vi "Calculate Analyte Yield.vi"(10 "Max Concentration":dbl, 11 "Peaks":string[][](array[string])) -> (3 "Yield out":dbl)   [LabVIEW 2020, in "Waters Patrol UPLC Report Parser.lvlib"]
uses:
  Waters Patrol UPLC Report Parser.lvlib
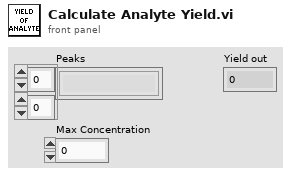
[diagram p1: front panel]
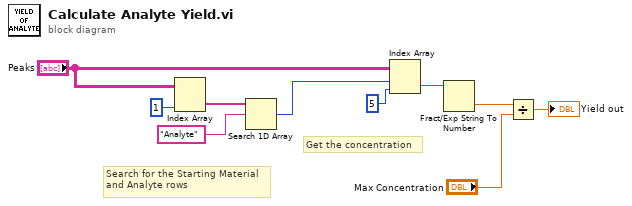
[diagram p0: block diagram]
diagram:
  # "Get the concentration"
  # "Search for the Starting Material\nand Analyte rows"
  n1 = Index Array(array="Peaks", index (col)=1 ("disabled index (col)")) -> (element=w6:string[])  [unwired: 1 in]
  n2 = Search 1D Array(1D array=w6, element="Analyte") -> (index of element=w8:i32)  [unwired: 1 in]
  n3 = Index Array(array="Peaks", index (row)=w8, index (col)=5 ("disabled index (col)")) -> (element=w7:string)
  n4 = Fract/Exp String To Number(string=w7) -> (number=w3:dbl)  [unwired: 3 in, 1 out]
  n5 = Divide(x=w3, y="Max Concentration") -> (x/y=→"Yield out":dbl)
